vi "BARCODE_SEARCH.vi"(8 "error in":errorcluster, 9 "BARCODE_TABLE":string[][](table), 11 "BARCODE_TO_SEARCH":string) -> (0 "error out":errorcluster, 1 "ARTICLE name":string, 2 "FOUND_ROW":string[](array[string]), 3 "BARCODE_FOUND":bool, 4 "description NAME":string, 5 "CHL":T1)   [LabVIEW 2017]
panel:
  out "CHL 3":T2
  out "CHL 2":T3
  out "CHL 1":T4
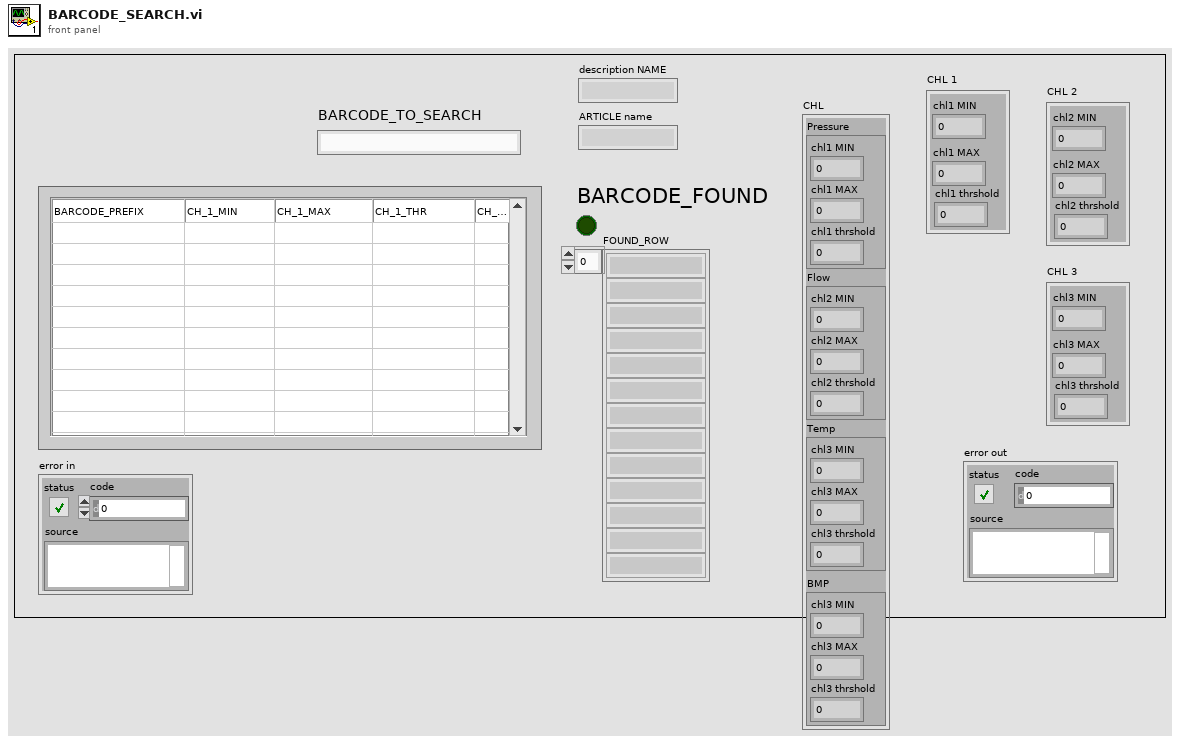
[diagram p1: front panel]
types:
  T1 = cluster{"Pressure":cluster{"chl1 MIN":dbl, "chl1 MAX":dbl, "chl1 thrshold":dbl}, "Flow":cluster{"chl2 MIN":dbl, "chl2 MAX":dbl, "chl2 thrshold":dbl}, "Temp":cluster{"chl3 MIN":dbl, "chl3 MAX":dbl, "chl3 thrshold":dbl}, "BMP":cluster{"chl3 MIN":dbl, "chl3 MAX":dbl, "chl3 thrshold":dbl}}
  T2 = cluster{"chl3 MIN":dbl, "chl3 MAX":dbl, "chl3 thrshold":dbl}
  T3 = cluster{"chl2 MIN":dbl, "chl2 MAX":dbl, "chl2 thrshold":dbl}
  T4 = cluster{"chl1 MIN":dbl, "chl1 MAX":dbl, "chl1 thrshold":dbl}
  T5 = cluster{"Pressure":cluster{"chl1 MIN":dbl, "chl1 MAX":dbl, "chl1 thrshold":dbl}, "Flow":cluster{"chl2 MIN":dbl, "chl2 MAX":dbl, "chl2 thrshold":dbl}, "Temp":cluster{"chl3 MIN":dbl, "chl3 MAX":dbl, "chl3 thrshold":dbl}, "BMP":cluster{"chl2 MIN":dbl, "chl2 MAX":dbl, "chl2 thrshold":dbl}}
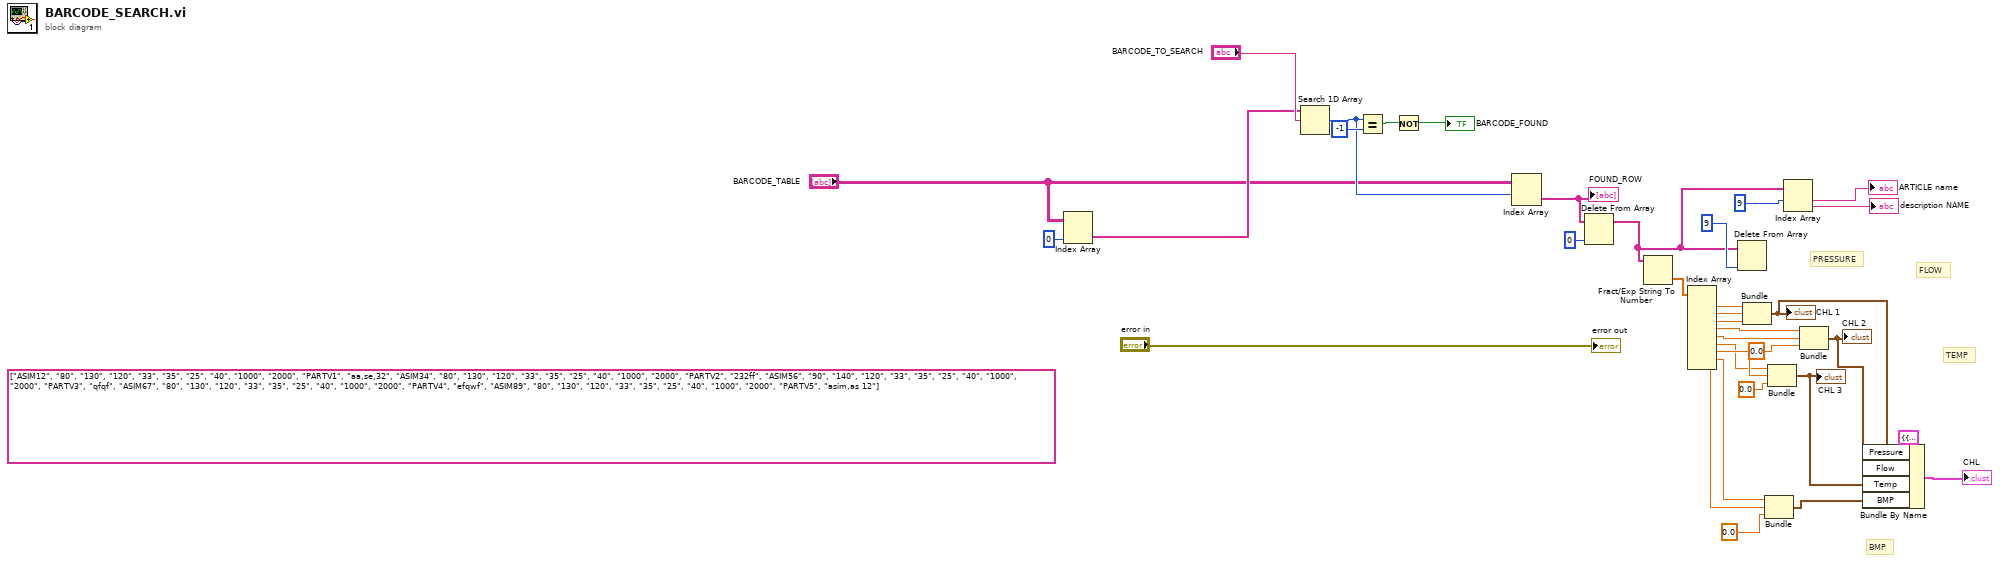
[diagram p0: block diagram]
diagram:
  (unwired) string[][] [["ASIM12", "80", "130", "120", "33", "35", "25", "40", "1000", "2000", "PARTV1", "aa,se,32"], ["ASIM34", "80", "130", "120", "33", "35", "25", "40", "1000", "2000", "PARTV2", "232ff"], ["ASIM56", "90", "140", "120", "33", "35", "25", "40", "1000", "2000", "PARTV3", "qfqf"], ["ASIM67", "80", "130", "120", "33", "35", "25", "40", "1000", "2000", "PARTV4", "efqwf"], ["ASIM89", "80", "130", "120", "33", "35", "25", "40", "1000", "2000", "PARTV5", "asim,as 12"]] ("table")
  # "BMP"
  # "TEMP"
  # "FLOW"
  # "PRESSURE"
  n1 = Index Array(array="BARCODE_TABLE", index (col)=0 ("disabled index (col)")) -> (element=w20:string[])  [unwired: 1 in]
  n2 = Search 1D Array(1D array=w20, element="BARCODE_TO_SEARCH") -> (index of element=w31:i32)  [unwired: 1 in]
  n3 = Equal?(x=w31, y=-1) -> (x = y?=w34:bool)
  n4 = Not(x=w34) -> (.not. x?=→"BARCODE_FOUND":bool)
  n5 = Index Array(array="BARCODE_TABLE", index (row)=w31) -> (element=w29:string[])  [unwired: 1 in]
  "FOUND_ROW" <- w29
  n6 = Delete From Array(array=w29, index=0) -> (array with subset deleted=w18:string[])  [unwired: 1 in, 1 out]
  n7 = Fract/Exp String To Number(string=w18) -> (number=w27:dbl[])  [unwired: 3 in, 1 out]
  n8 = Index Array(array=w27) -> (element #1=w24:dbl, element #2=w25:dbl, element #3=w26:dbl, element #4=w23:dbl, element #5=w22:dbl, element #6=w6:dbl, element #7=w7:dbl, element #8=w4:dbl, element #9=w3:dbl)  [unwired: 9 in]
  n9 = Delete From Array(array=w18, index=9) -> ()  [unwired: 1 in, 2 out]
  n10 = Bundle(w24, w25, w26) -> (w14:cluster{dbl, dbl, dbl})  [unwired: 1 in]
  "CHL 1" <- w14
  n11 = Bundle(w4, w3, "element"=0.0) -> (w5:cluster{dbl, dbl, "element":dbl})  [unwired: 1 in]
  n12 = Bundle(w6, w7, "element"=0.0) -> (w12:cluster{dbl, dbl, "element":dbl})  [unwired: 1 in]
  "CHL 3" <- w12
  n13 = Index Array(array=w18, index #1=9 ("index")) -> (element #1=→"ARTICLE name":string, element #2=→"description NAME":string)  [unwired: 1 in]
  n14 = Bundle(w23, w22, "element"=0.0) -> (w13:cluster{dbl, dbl, "element":dbl})  [unwired: 1 in]
  "CHL 2" <- w13
  n15 = Bundle By Name(cluster=T5 {"Pressure"={"chl1 MIN"=110.0, "chl1 MAX"=130.0, "chl1 thrshold"=120.0}, "Flow"={"chl2 MIN"=33.0, "chl2 MAX"=35.0, "chl2 thrshold"=25.0}, "Temp"={"chl3 MIN"=20.0, "chl3 MAX"=30.0, "chl3 thrshold"=34.0}, "BMP"={"chl2 MIN"=33.0, "chl2 MAX"=35.0, "chl2 thrshold"=25.0}}, "Pressure"=w14, "Flow"=w13, "Temp"=w12, "BMP"=w5) -> (→"CHL":T5)
  "error out" <- "error in"
